vi "脉冲生成_基于时钟滴答_连续.vi"() -> ()   [LabVIEW 2013]
uses:
  <userlib>/ArtDAQ/_SubVI/ArtDAQ_CreateCOPulseChanTicks.vi
  <userlib>/ArtDAQ/_SubVI/ArtDAQ_CfgImplicitTiming.vi
  <userlib>/ArtDAQ/_SubVI/ArtDAQ_CfgDigEdgeStartTrig.vi
  <userlib>/ArtDAQ/_SubVI/ArtDAQ_CfgDigLvlPauseTrig.vi
panel:
  in  "时钟滴答源":string="/Dev1/PFI1"
  in  "TriggerMode":T1(tab)
  in  "触发边沿":i32(ring)=10280 items=["上升"=10280, "下降"=10171]
  in  "触发源":string(combo)="/Dev1/PFI2"
  in  "触发源":string="/Dev1/PFI2"
  in  "暂停条件":i32(ring)=10192 items=["高"=10192, "低"=10214]
  in  "每通道采样":i32=1000
  in  "Stop":bool
  in  "计数器":string="Dev1/ctr0"
  in  "高滴答数":i32=100
  in  "低滴答数":i32=100
  out "错误输出":errorcluster
  # "通道属性"
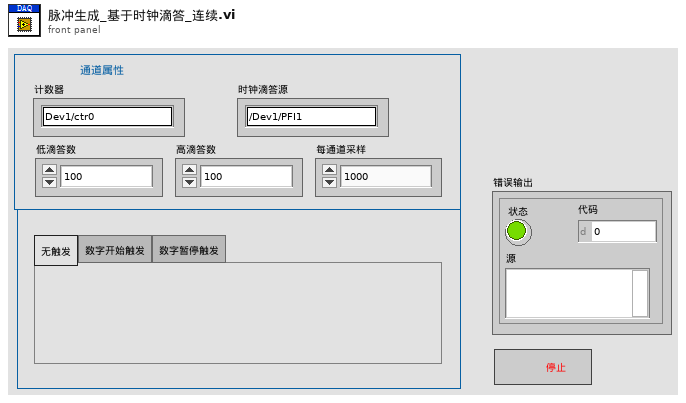
[diagram p1: front panel]
types:
  T1 = enum32{"No Trigger", "DigStartTrig", "DigPauseTrig"}
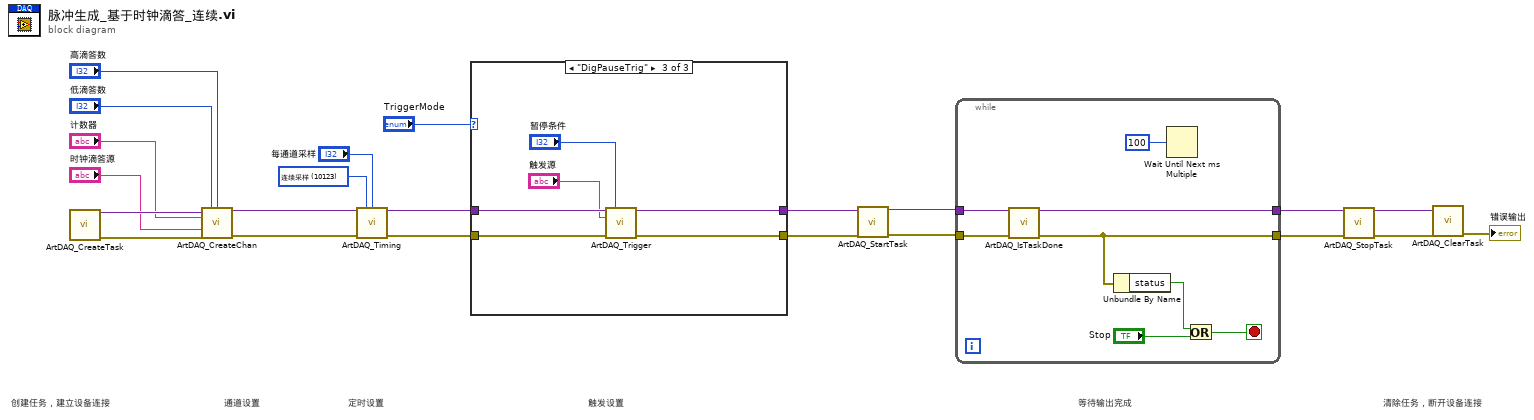
[diagram p0: block diagram]
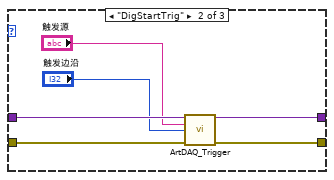
[diagram p3: hidden frame]
diagram:
  w11 = 10123 items=["有限点采样"=10178, "连续采样"=10123] ("SampleMode")
  # "清除任务，断开设备连接"
  # "等待输出完成"
  # "定时设置"
  # "触发设置"
  # "通道设置"
  # "创建任务，建立设备连接"
  n1 = call <userlib>:"ArtDAQ_CreateTask.vi"() -> ("任务句柄"=w22:variant, "错误输出"=w21:errorcluster)  [unwired: 14 in]
  n2 = call-poly <userlib>:"ArtDAQ_CreateChan.vi"("任务句柄"=w22, "低时钟滴答"="低滴答数", "高时钟滴答"="高滴答数", "计数器"="计数器", "时钟滴答源"="时钟滴答源", "错误输入"=w21) -> ("任务句柄"=w13:variant, "错误输出"=w12:errorcluster)  [unwired: 8 in]
  n3 = call-poly <userlib>:"ArtDAQ_Timing.vi"("任务句柄"=w13, "采样模式"=w11, "每通道采样数"="每通道采样", "错误输入"=w12) -> ("任务句柄"=w8:variant, "错误输出"=w7:errorcluster)  [unwired: 10 in]
  n4 = case shown="\"DigPauseTrig\"" "TriggerMode" {
    tunnel: w8 -> [w24 w30 w36]
    tunnel: [w24 w29 w35] -> w6
    tunnel: [w23 w28 w33] -> w4
    tunnel: w7 -> [w23 w27 w34]
    frame "No Trigger", Default {
    }
    frame "DigStartTrig" {
      n5 = call-poly <userlib>:"ArtDAQ_Trigger.vi"("任务句柄"=w30, "触发源"="触发源", "边沿"="触发边沿", "错误输入"=w27) -> ("任务句柄"=w29:variant, "错误输出"=w28:errorcluster)  [unwired: 10 in]
    }
    frame "DigPauseTrig" {
      n6 = call-poly <userlib>:"ArtDAQ_Trigger.vi"("任务句柄"=w36, "触发条件"="暂停条件", "触发源"="触发源", "错误输入"=w34) -> ("任务句柄"=w35:variant, "错误输出"=w33:errorcluster)  [unwired: 10 in]
    }
  }
  n7 = call <userlib>:"ArtDAQ_StartTask.vi"("任务句柄"=w6, "错误输入"=w4) -> ("任务句柄"=w5:variant, "错误输出"=w3:errorcluster)  [unwired: 12 in]
  n8 = while {
    tunnel: [w44] -> w20
    tunnel: [w43] -> w18
    tunnel: w5 -> [w40]
    tunnel: w3 -> [w39]
    stop <- w38 stop-if-true
    n9 = call <userlib>:"ArtDAQ_IsTaskDone.vi"("任务句柄"=w40, "错误输入"=w39) -> ("任务句柄"=w44:variant, "错误输出"=w43:errorcluster)  [unwired: 11 in, 1 out]
    n10 = Unbundle By Name(w43) -> ("status"=w42:bool)
    n11 = Wait Until Next ms Multiple(millisecond multiple=u32 100 ("毫秒倍数")) -> ()  [unwired: 1 out]
    n12 = Or(x=w42, y="Stop") -> (x .or. y?=w38:bool)
  }
  n13 = call <userlib>:"ArtDAQ_StopTask.vi"("任务句柄"=w20, "错误输入"=w18) -> ("任务句柄"=w19:variant, "错误输出"=w17:errorcluster)  [unwired: 12 in]
  n14 = call <userlib>:"ArtDAQ_ClearTask.vi"("任务句柄"=w19, "错误输入"=w17) -> ("错误输出"=→"错误输出":errorcluster)  [unwired: 13 in]
